vi "Decode uint32.vi"(10 "Wire Type":T1, 11 "Data":u8[](array[numeric]) format="%.0x") -> (2 "error out":errorcluster, 3 "uint32":u32)   [LabVIEW 2020, in "LV-Proto.lvlib"]
uses:
  LV-Proto.lvlib
  Wire Type.ctl
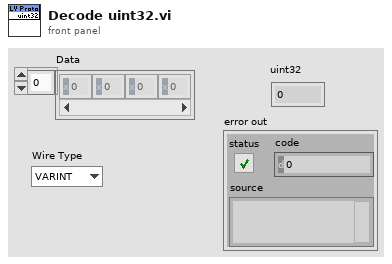
[diagram p1: front panel]
types:
  T1 = typedef "LV-Proto.lvlib/Wire Type.ctl" = enum8{"VARINT", "I64", "LEN", "SGROUP (Deprecated)", "EGROUP (Deprecated)", "I32"}
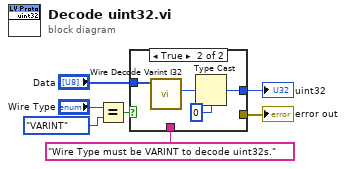
[diagram p0: block diagram]
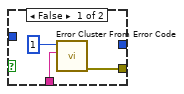
[diagram p2: hidden frame]
diagram:
  n1 = Equal?(x="Wire Type", y=Wire_Type."VARINT") -> (x = y?=w3:bool)
  n2 = case shown="True" w3 {
    tunnel: [_ w11] -> w7
    tunnel: "Data" -> [_ w14]
    tunnel: [w9 _] -> w2
    tunnel: "Wire Type must be VARINT to decode uint32s." -> [w8 _]
    frame False {
      n3 = call <vilib>:"Error Cluster From Error Code.vi"("error message (\"\")"=w8, "error code (0)"=1) -> ("error out"=w9:errorcluster)  [unwired: 7 in]
    }
    frame True {
      n4 = call "Wire Decode Varint I32.vi"("Buffer in"=w14) -> ("I32"=w13:i32)  [unwired: 9 in, 1 out]
      n5 = Type Cast(type=u32 0, x=w13) -> (*(type *) &x=w11:u32)
    }
  }
  "uint32" <- w7
  "error out" <- w2
